vi "Exponential Fit Coefficients (Bisquare).vi"(0 "Y":dbl[](array[numeric]), 5 "X":dbl[](array[numeric]), 7 "Weight":dbl[](array[numeric]), 9 "tolerance":dbl=0.0001 format="%#_3g", 11 "Initial Coefficients":dbl[](array[numeric]), 12 "algorithm":u16(ring) items=["Semi-Log", "Iterative"]) -> (4 "amplitude":dbl, 6 "damping":dbl, 15 "error":i32)   [LabVIEW 2010, in "NI_AALPro.lvlib"]
uses:
  NI_AALPro.lvlib
  lvanlys.dll
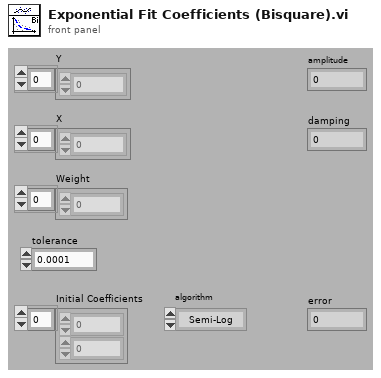
[diagram p1: front panel]
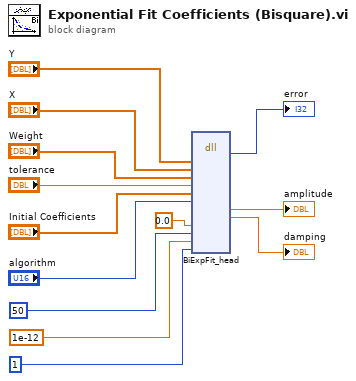
[diagram p0: block diagram]
diagram:
  n1 = dll-call lib="C:/Program Files/National Instruments/LabVIEW 2010/resource/lvanlys.*" fn="BiExpFit_head"("y"="Y", "x"="X", "weight"="Weight", "tolerance"="tolerance", "intial coef"="Initial Coefficients", "algorithm"="algorithm", "mearErr"=0.0, "maxIter"=50, "absTol"=1e-12, "isCoef"=1 ("maxIter")) -> (→"error":i32, "amp"=→"amplitude":dbl, "damping"=→"damping":dbl)  [unwired: 15 in, 2 out]
